vi "E8267D SetPower.vi"(0 "VISA Rsrc":refnum<visa-resource-name>="GPIB0::12::INSTR", 5 "Power dBm":dbl, 11 "error in (no error)":errorcluster) -> (4 "VISA Rsrc Out":refnum<visa-resource-name>="GPIB0::12::INSTR", 15 "error out":errorcluster)   [LabVIEW 2019]
doc: "Ce VI écrit les paramètres de la zone de contrôle spécifiée dans le contrôlleur"
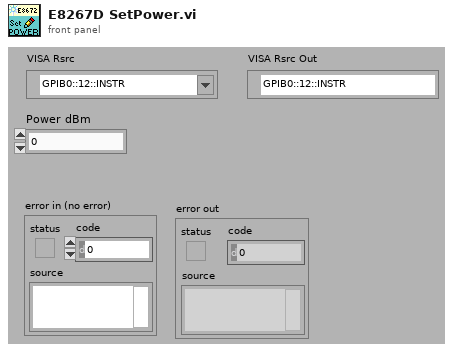
[diagram p1: front panel]
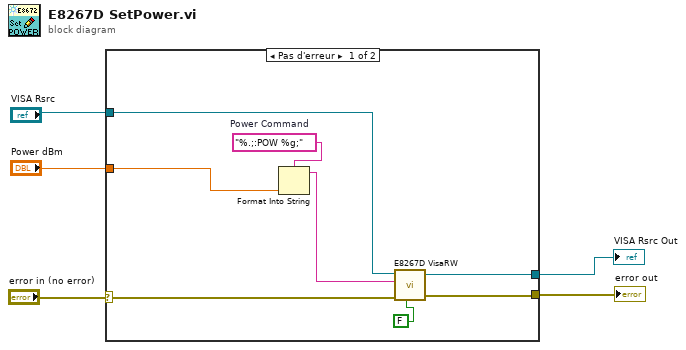
[diagram p0: block diagram]
diagram:
  n1 = case shown="Pas d'erreur" "error in (no error)" {
    selector: "error in (no error)" -> [w12 w15]
    tunnel: "VISA Rsrc" -> [w11 w14]
    tunnel: [w13 w15] -> w4
    tunnel: "Power dBm" -> [w8 _]
    tunnel: [w9 w14] -> w1
    frame No Error {
      w6 = "%.;:POW %g;"  # Power Command
      n2 = Format Into String(format string=w6, w8) -> (resulting string=w7:string)  [unwired: 2 in, 1 out]
      n3 = call <userlib>:"E8267D VisaRW.vi"("Lecture?(T)"=FALSE, "error in (no error)"=w12, "ChaineCom"=w7, "VISA Rsrc"=w11) -> ("error out"=w13:errorcluster, "VISA Rsrc Out"=w9:refnum<visa-resource-name>)  [unwired: 3 in, 2 out]
    }
    frame Error {
    }
  }
  "error out" <- w4
  "VISA Rsrc Out" <- w1
